vi "CAM_pp3c_display.vi"(8 "Camera":T1="cam0", 9 "Log File Directory":refnum<vi>, 10 "Loop state Refnum":refnum<vi>, 11 "Image Ctl Refnum":refnum<vi>) -> ()   [LabVIEW 2013]
doc: "This VI is a general VI that loops through webcam images, and saves when necessary. It should be run asynchronously, so that webcam display/logging is independent of the main loop. Terminate this VI by setting the \"Webcam on\" value within the state info refnum to False."
uses:
  <vilib>/vision/driver/NI_Vision_Acquisition_Software.lvlib
  <vilib>/vision/Image Controls.llb/IMAQ Image.ctl
  <vilib>/userdefined/High Color/IMAQdx.ctl
  CTL_pp3c_LoopState.ctl
  pp3_CTL_BehavioralState.ctl
  pp3_CTL_Trial.ctl
  pp3_CTL_TrialType.ctl
  labolabo2/waveforms/WFTypes.ctl
panel:
  out "error out":errorcluster
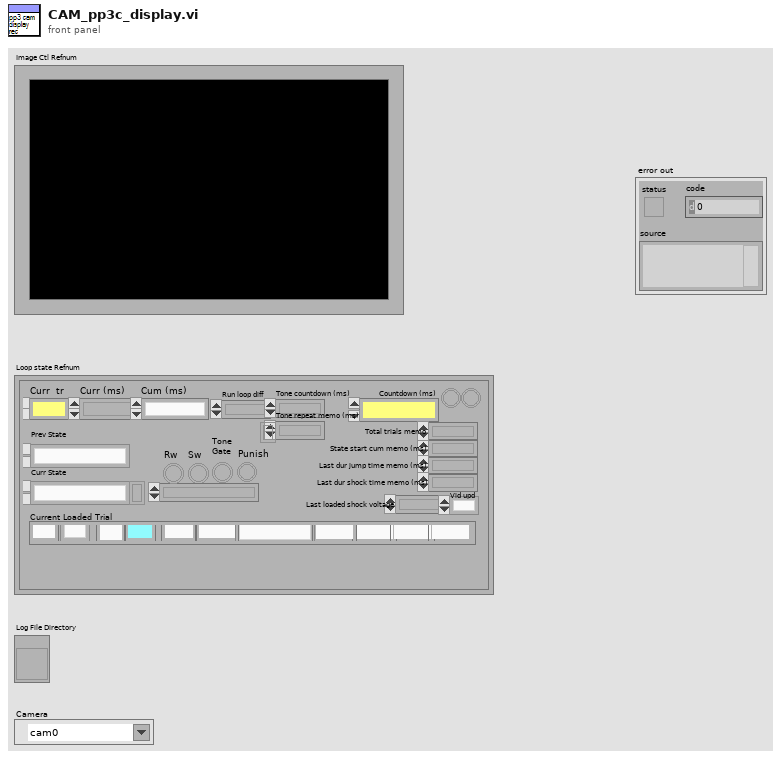
[diagram p1: front panel]
types:
  T1 = typedef "IMAQdx.ctl" = refnum<k21>
  T2 = typedef "CTL_pp3c_LoopState.ctl" = cluster{"Curr  tr":u16, "Curr (ms)":u32, "Cum (ms)":u64, "Run loop diff":i64, "Tone countdown (ms)":i64, "Countdown (ms)":i64, "Curr State":T3, "Prev State":T3, "Rw":bool, "Sw":bool, "Tone\nGate":bool, "Punish":bool, "Current DAQ DO Int":u16, "Current Loaded Trial":T4, "Total trials memo":i64, "State start cum memo (ms)":i64, "Last dur jump time memo (ms)":i64, "Last dur shock time memo (ms)":i64, "Tone repeat memo (ms)":i64, "Webcam on":bool, "Webcam recording":bool, "State update flag":bool, "Last loaded shock voltage":dbl, "Vid upd":enum16{"0", "1", "2", "3", "4", "5", "6", "7", "8", "9"}, "First time tone":bool}
  T3 = typedef "pp3_CTL_BehavioralState.ctl" = enum8{"0 NULL", "1 Habituation", "2 (Load Trial)", "3 Stay Period", "4 Load Audio/Click Delay", "5 GO Trial", "6 GO Jumped", "7 GO Timeout", "8 NOGO Trial", "9 NOGO Jumped", "10 NOGO Timeout", "11 TEST Trial", "12 TEST Jumped", "13 TEST Timeout", "14 Intertrial Interval", "15 Done"}
  T4 = typedef "pp3_CTL_Trial.ctl" = cluster{"Trial Type Number":i16, "Trial Type":T5, "Trial Weight":u32, "Shock (mA)":dbl, "Duration (ms)":dbl, "Sound Type":T6, "Stim P1":dbl, "Stim P2":dbl, "Stim P3":dbl, "Stim P4":dbl, "DAQ Amplitude (V)":dbl}
  T5 = typedef "pp3_CTL_TrialType.ctl" = enum16{"OFF", "GO", "NOGO", "TEST"}
  T6 = typedef "WFTypes.ctl" = enum16{"00 NULL", "01 DC", "02 Noise", "03 Pure Tone", "04 FM Sweep"}
  T7 = typedef "IMAQ Image.ctl" = refnum<image>
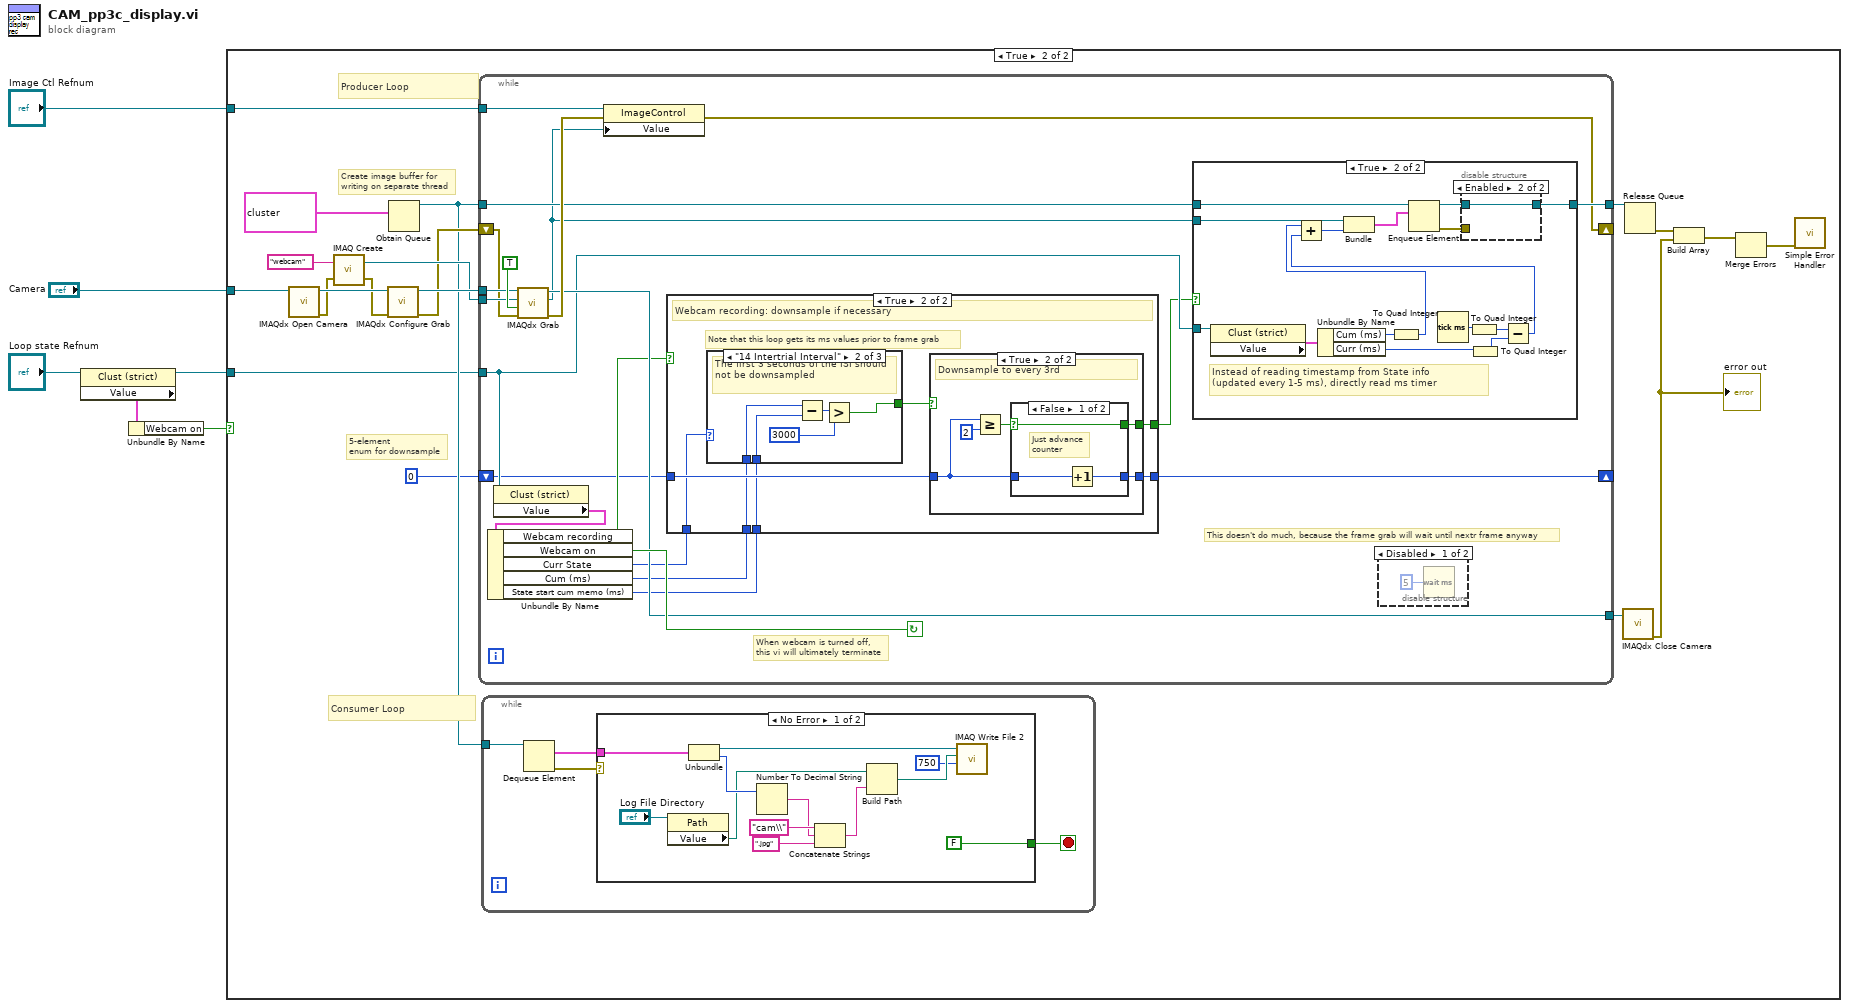
[diagram p0: block diagram]
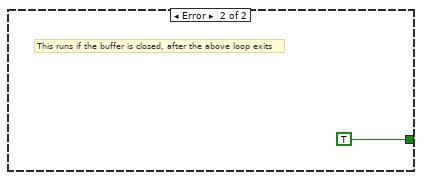
[diagram p3: hidden frame]
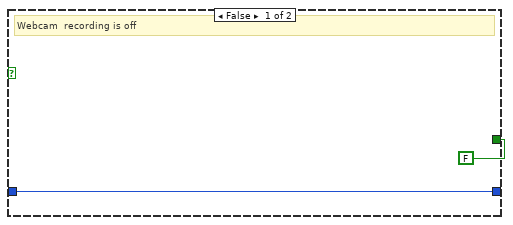
[diagram p5: hidden frame]
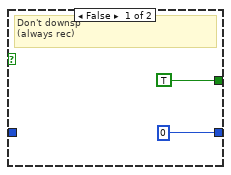
[diagram p6: hidden frame]
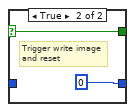
[diagram p7: hidden frame]
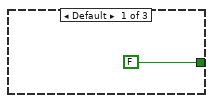
[diagram p8: hidden frame]
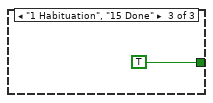
[diagram p9: hidden frame]
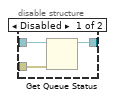
[diagram p11: hidden frame]
diagram:
  n1 = property class="Clust (strict)"(reference="Loop state Refnum") -> (reference out=w3:refnum<vi>, "Value"=w2:T2)  [unwired: 1 in, 1 out]
  n2 = Unbundle By Name(w2) -> ("Webcam on"=w1:bool)
  n3 = case shown="True" w1 {
    tunnel: "Image Ctl Refnum" -> [_ w25]
    tunnel: "Camera" -> [_ w21]
    tunnel: w3 -> [_ w8]
    frame False {
    }
    frame True {
      # "Consumer Loop"
      # "Producer Loop"
      # "5-element\nenum for downsample"
      # "Create image buffer for\nwriting on separate thread"
      n4 = call <vilib>:"IMAQdx Open Camera.vi"("Session In"=w21) -> ("error out"=w20:errorcluster, "Session Out"=w23:T1)  [unwired: 9 in]
      n5 = call "IMAQ Create"("Image Name"="webcam", "error in (no error)"=w20) -> ("New Image"=w17:T7, "error out"=w19:errorcluster)  [unwired: 3 in]
      n6 = call <vilib>:"IMAQdx Configure Grab.vi"("error in"=w19, "Session In"=w23) -> ("error out"=w11:errorcluster, "Session Out"=w18:T1)  [unwired: 8 in]
      n7 = Obtain Queue(element data type=cluster{"Image":T7, "Cum (ms)":i64} {"Image"="Webcam", "Cum (ms)"=0}) -> (queue out=w9:refnum<queue>)  [unwired: 4 in, 2 out]
      n8 = while {
        tunnel: w18 -> [w60]
        tunnel: w17 -> [w59]
        tunnel: w9 -> [w58]
        tunnel: [w56] -> w16
        tunnel: [w55] -> w12
        shift-right: [w52] -> _
        shift-left: w11 -> [w54]
        tunnel: w8 -> [w51]
        tunnel: w25 -> [w62]
        shift-right: [w46] -> _
        shift-left: 0 -> [w48]
        stop <- w57 continue-if-true
        # "This doesn't do much, because the frame grab will wait until nextr frame anyway"
        # "When webcam is turned off,\nthis vi will ultimately terminate"
        n9 = property class="Clust (strict)"(reference=w51) -> ("Value"=w49:T2)  [unwired: 1 in, 2 out]
        n10 = Unbundle By Name(w49) -> ("Webcam recording"=w50:bool, "Webcam on"=w57:bool, "Curr State"=w45:T3, "Cum (ms)"=w44:u64, "State start cum memo (ms)"=w43:i64)
        n11 = call <vilib>:"IMAQdx Grab.vi"("error in"=w54, "Wait for Next Buffer? (Yes)"=TRUE, "Image In"=w59, "Session In"=w60) -> ("error out"=w63:errorcluster, "Image Out"=w53:T7, "Session Out"=w56:T1)  [unwired: 4 in, 1 out]
        n12 = property class="ImageControl"(reference=w62, error in=w63, "Value"=w53) -> (error out=w52:errorcluster)  [unwired: 1 out]
        n13 = case shown="True" w50 {
          tunnel: w48 -> [w65 w70]
          tunnel: [FALSE w72] -> w47
          tunnel: [w65 w71] -> w46
          tunnel: w45 -> [_ w69]
          tunnel: w44 -> [_ w68]
          tunnel: w43 -> [_ w67]
          frame False {
            # "Webcam  recording is off"
          }
          frame True {
            # "Note that this loop gets its ms values prior to frame grab"
            # "Webcam recording: downsample if necessary"
            n14 = case shown="\"14 Intertrial Interval\"" w69 {
              tunnel: [FALSE w89 TRUE] -> w73
              tunnel: w68 -> [_ w88 _]
              tunnel: w67 -> [_ w87 _]
              frame Default {
              }
              frame "14 Intertrial Interval" {
                # "The first 3 seconds of the ISI should not be downsampled"
                n15 = Subtract(x=w88, y=w87) -> (x-y=w91:u64)
                n16 = Greater?(x=w91, y=i64 3000) -> (0:w89:bool)
              }
              frame "1 Habituation", "15 Done" {
              }
            }
            n17 = case shown="True" w73 {
              tunnel: [TRUE w76] -> w72
              tunnel: [0 w78] -> w71
              tunnel: w70 -> [_ w77]
              frame False {
                # "Don't downsp\n(always rec)"
              }
              frame True {
                # "Downsample to every 3rd"
                n18 = Greater Or Equal?(x=w77, y=2) -> (x >= y?=w79:bool)
                n19 = case shown="False" w79 {
                  selector: w79 -> [w81 w85]
                  tunnel: [w83 0] -> w78
                  tunnel: w77 -> [w82 _]
                  tunnel: [w81 w85] -> w76
                  frame False {
                    # "Just advance\ncounter"
                    n20 = Increment(x=w82) -> (x+1=w83:i32)
                  }
                  frame True {
                    # "Trigger write image\nand reset"
                  }
                }
              }
            }
          }
        }
        n21 = case shown="True" w47 {
          tunnel: w53 -> [_ w109]
          tunnel: w58 -> [w93 w108]
          tunnel: [w93 w106] -> w55
          tunnel: w51 -> [_ w104]
          frame False {
          }
          frame True {
            # "Instead of reading timestamp from State info\n(updated every 1-5 ms), directly read ms timer"
            n22 = property class="Clust (strict)"(reference=w104) -> ("Value"=w103:T2)  [unwired: 1 in, 2 out]
            n23 = Unbundle By Name(w103) -> ("Cum (ms)"=w95:u64, "Curr (ms)"=w99:u32)
            n24 = To Quad Integer(1:w95) -> (0:w94:i64)
            n25 = Tick Count (ms)() -> (millisecond timer value=w97:u32)
            n26 = To Quad Integer(1:w97) -> (0:w96:i64)
            n27 = To Quad Integer(1:w99) -> (0:w98:i64)
            n28 = Subtract(x=w96, y=w98) -> (x-y=w100:i64)
            n29 = Add(x=w94, y=w100) -> (x+y=w101:i64)
            n30 = Bundle("Image Out"=w109, w101) -> (w102:cluster{"Image Out":T7, i64})  [unwired: 1 in]
            n31 = Enqueue Element(queue=w108, element=w102) -> (queue out=w107:refnum<queue>, error out=w105:errorcluster)  [unwired: 2 in, 1 out]
            n32 = disable-structure shown="Enabled" {
              disable-tunnel: w107 -> [w112 w113]
              disable-tunnel: [w111 w113] -> w106
              disable-tunnel: w105 -> [w110 _]
              frame Disabled {
                n33 = Get Queue Status(queue=w112, error in (no error)=w110) -> (queue out=w111:refnum<queue>)  [unwired: 1 in, 7 out]
              }
              frame Enabled {
              }
            }
          }
        }
        n34 = disable-structure shown="Disabled" {
          frame Disabled {
            n35 = Wait (ms)(milliseconds to wait=u32 5) -> ()  [unwired: 1 out]
          }
          frame Enabled {
          }
        }
      }
      n36 = while {
        tunnel: w9 -> [w29]
        stop <- w27 stop-if-true
        n37 = Dequeue Element(queue=w29) -> (element=w26:cluster{"Image":T7, "Cum (ms)":i64}, error out=w28:errorcluster)  [unwired: 2 in, 2 out]
        n38 = case shown="No Error" w28 {
          tunnel: [FALSE TRUE] -> w27
          tunnel: w26 -> [w40 _]
          frame No Error {
            n39 = property class="Path"(reference="Log File Directory") -> ("Value"=w31:path)  [unwired: 1 in, 2 out]
            n40 = Unbundle(w40) -> ("Image"=w33:T7, "Cum (ms)"=w37:i64)
            n41 = Number To Decimal String(number=w37) -> (decimal integer string=w36:string)  [unwired: 1 in]
            n42 = Concatenate Strings("cam\\", w36, ".jpg" ("string")) -> (w35:string)
            n43 = Build Path(base path=w31, name or relative path=w35) -> (appended path=w34:path)
            n44 = call-poly "IMAQ Write File 2"("Image Quality"=u32 750, "File Path"=w34, "Image"=w33) -> ()  [unwired: 7 in, 2 out]
          }
          frame Error {
            # "This runs if the buffer is closed, after the above loop exits"
          }
        }
      }
      n45 = call <vilib>:"IMAQdx Close Camera.vi"("Session In"=w16) -> ("error out"=w10:errorcluster)  [unwired: 10 in]
      "error out" <- w10
      n46 = Release Queue(queue=w12) -> (error out=w15:errorcluster)  [unwired: 2 in, 2 out]
      n47 = Build Array(w15, w10) -> (w13:errorcluster[])
      n48 = Merge Errors(w13) -> (w14:errorcluster)  [unwired: 2 in]
      n49 = call <vilib>:"Simple Error Handler.vi"("error in (no error)"=w14) -> ()  [unwired: 4 in, 5 out]
    }
  }
